vi "SetAuxFeederSpeedDmd.vi"(11 "Feeder Demand":dbl) -> ()   [LabVIEW 2020]
uses:
  AuxGlobals.vi
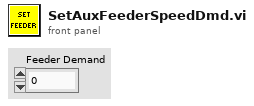
[diagram p1: front panel]
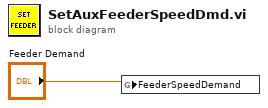
[diagram p0: block diagram]
diagram:
  n1 = global write "AuxGlobals.vi" "FeederSpeedDemand"("Feeder Demand") -> ()
